vi "linear_activation_forward.vi"(2 "activation":enum16{"sigmoid", "relu"}(ring), 3 "b":dbl[][](array[numeric]), 4 "W":dbl[][](array[numeric]), 5 "A_prev":dbl[][](array[numeric])) -> (0 "cache":T1, 1 "A":dbl[][](array[numeric]))   [LabVIEW 2020]
uses:
  Sigmoid.vi
  Relu.vi
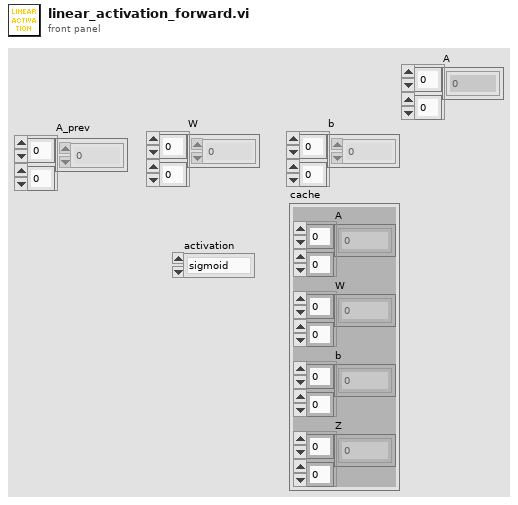
[diagram p1: front panel]
types:
  T1 = cluster{"A":dbl[][], "W":dbl[][], "b":dbl[][], "Z":dbl[][]}
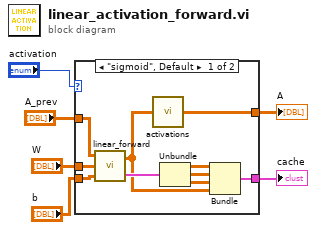
[diagram p0: block diagram]
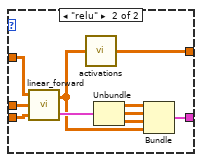
[diagram p2: hidden frame]
diagram:
  n1 = case shown="\"sigmoid\", Default" "activation" {
    tunnel: "b" -> [w14 w24]
    tunnel: "W" -> [w15 w25]
    tunnel: "A_prev" -> [w16 w26]
    tunnel: [w13 w23] -> w1
    tunnel: [w7 w17] -> w2
    frame "sigmoid", Default {
      n2 = call "linear_forward.vi"("b"=w14, "W"=w15, "A"=w16) -> ("cache"=w12:cluster{"A":dbl[][], "W":dbl[][], "b":dbl[][]}, "Z"=w8:dbl[][])
      n3 = call-poly "activations.vi"("Z"=w8) -> ("Sigmoid(Z)"=w13:dbl[][])  [unwired: 2 in]
      n4 = Unbundle(w12) -> ("A"=w11:dbl[][], "W"=w10:dbl[][], "b"=w9:dbl[][])
      n5 = Bundle("A"=w11, "W"=w10, "b"=w9, "Z"=w8) -> (w7:T1)  [unwired: 1 in]
    }
    frame "relu" {
      n6 = call "linear_forward.vi"("b"=w24, "W"=w25, "A"=w26) -> ("cache"=w22:cluster{"A":dbl[][], "W":dbl[][], "b":dbl[][]}, "Z"=w18:dbl[][])
      n7 = call-poly "activations.vi"("Z"=w18) -> ("Relu(Z)"=w23:dbl[][])  [unwired: 2 in]
      n8 = Unbundle(w22) -> ("A"=w21:dbl[][], "W"=w20:dbl[][], "b"=w19:dbl[][])
      n9 = Bundle("A"=w21, "W"=w20, "b"=w19, "Z"=w18) -> (w17:T1)  [unwired: 1 in]
    }
  }
  "cache" <- w2
  "A" <- w1
